vi "Wait_For_Position.vi"() -> ()   [LabVIEW 2018]
panel:
  in  "Node/Position Pairs":i64[][](array[numeric])
  out "Serial Out":refnum<visa-resource-name>
  out "Error Out":errorcluster
  in  "Error In":errorcluster
  in  "Serial In":refnum<visa-resource-name>
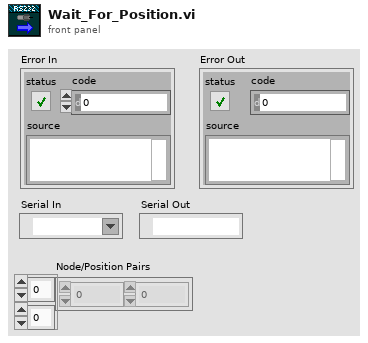
[diagram p1: front panel]
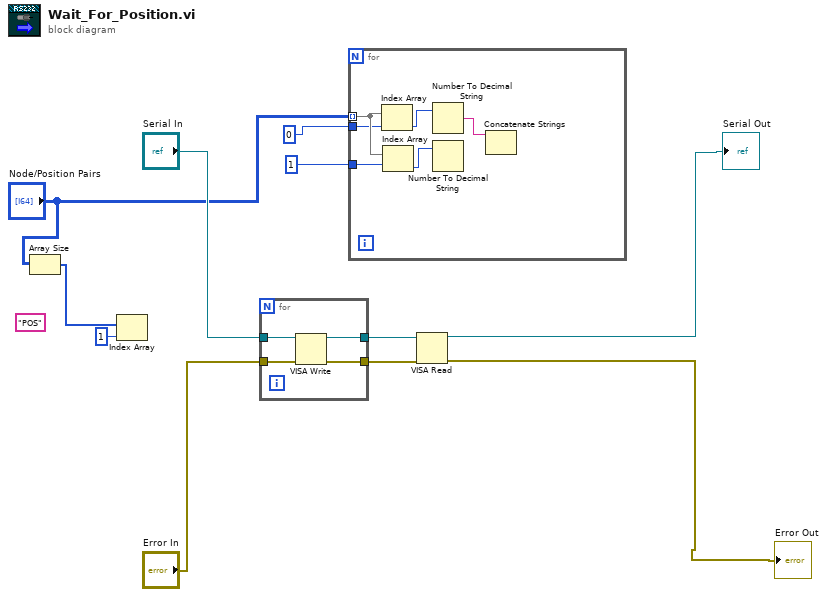
[diagram p0: block diagram]
diagram:
  (unwired) "POS"
  n1 = Array Size(array="Node/Position Pairs") -> (size(s)=w5:i32[])
  n2 = Index Array(array=w5, index=1) -> ()  [unwired: 1 out]
  n3 = for {
    tunnel: "Error In" -> [w15]
    tunnel: "Serial In" -> [w14]
    tunnel: [w13] -> w9
    tunnel: [w12] -> w8
    n4 = VISA Write(VISA resource name=w14, error in (no error)=w15) -> (VISA resource name out=w13:refnum<visa-resource-name>, error out=w12:errorcluster)  [unwired: 1 in, 1 out]
  }
  n5 = for {
    tunnel: "Node/Position Pairs" -> [w21] mode=indexing
    tunnel: 0 ("index") -> [w20]
    tunnel: 1 ("index") -> [w19]
    n6 = Index Array(array=w21, index=w20) -> (element=w18:i64)
    n7 = Index Array(array=w21, index=w19) -> (element=w17:i64)
    n8 = Number To Decimal String(number=w18) -> (decimal integer string=w16:string)  [unwired: 1 in]
    n9 = Number To Decimal String(number=w17) -> ()  [unwired: 1 in, 1 out]
    n10 = Concatenate Strings(w16) -> ()  [unwired: 2 in, 1 out]
  }
  n11 = VISA Read(VISA resource name=w9, error in (no error)=w8) -> (VISA resource name out=→"Serial Out":refnum<visa-resource-name>, error out=→"Error Out":errorcluster)  [unwired: 1 in, 2 out]
